vi "Log.vi"(8 "error in (no error)":errorcluster, 10 "Log Text":string, 11 "G-CLI Sink in":refnum<class "G-CLI Sink.lvclass">) -> (0 "error out":errorcluster, 3 "G-CLI Sink out":refnum<class "G-CLI Sink.lvclass">)   [LabVIEW 2020, in "LV Log.lvlib" / "G-CLI Sink.lvclass"]
uses:
  G-CLI Sink.lvclass
  G-CLI Sink.lvclass/G-CLI Sink.ctl
  <vilib>/Wiresmith Technology/G CLI/CLI Class/CLI.lvclass
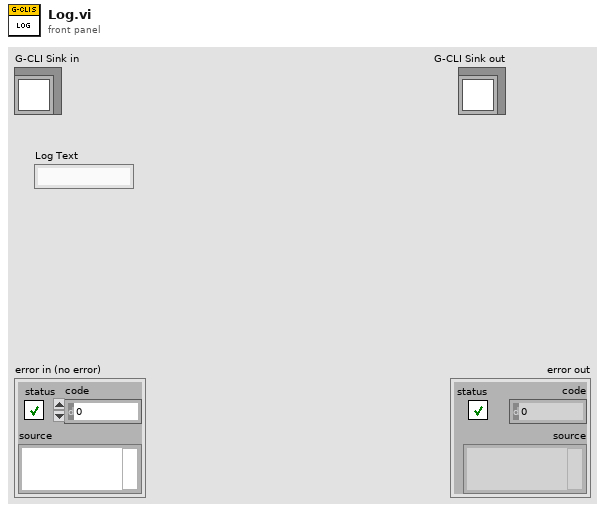
[diagram p1: front panel]
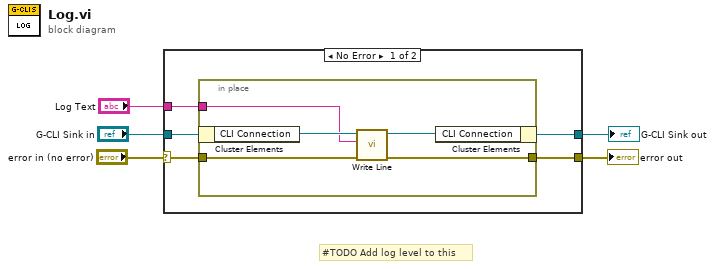
[diagram p0: block diagram]
diagram:
  # "#TODO Add log level to this"
  n1 = case shown="No Error" "error in (no error)" {
    selector: "error in (no error)" -> [w8 w16]
    tunnel: "G-CLI Sink in" -> [w10 w17]
    tunnel: [w9 w17] -> w3
    tunnel: [w7 w16] -> w2
    tunnel: "Log Text" -> [w6 _]
    frame No Error {
      n2 = in-place {
        in-place-border: w8 -> [w13]
        in-place-border: [w12] -> w7
        in-place-border: w6 -> [w11]
        n3 = in-place-cluster #1(w10) -> ("CLI Connection"=w15:refnum<class "CLI.lvclass">)
        n4 = call <vilib>:"Write Line.vi"("error in (no error)"=w13, "Text to Write"=w11, "CLI in"=w15) -> ("error out"=w12:errorcluster, "CLI out"=w14:refnum<class "CLI.lvclass">)  [unwired: 7 in]
        n5 = in-place-cluster #1("CLI Connection"=w14) -> (w9:refnum<class "G-CLI Sink.lvclass">)
      }
    }
    frame Error {
    }
  }
  "error out" <- w2
  "G-CLI Sink out" <- w3
